vi "Begin Transaction.vi"(8 "error in (no error)":errorcluster, 11 "Sqlite Database Manager in":refnum<class "Sqlite Database Manager.lvclass">) -> (0 "error out":errorcluster, 3 "Sqlite Database Manager out":refnum<class "Sqlite Database Manager.lvclass">)   [LabVIEW 2019, in "HierDAL Library.lvlib" / "Database.lvlib" / "Sqlite Database Manager.lvclass"]
uses:
  Sqlite Database Manager.lvclass
  Sqlite Database Manager.lvclass/Sqlite Database Manager.ctl
  System.Data.SQLite
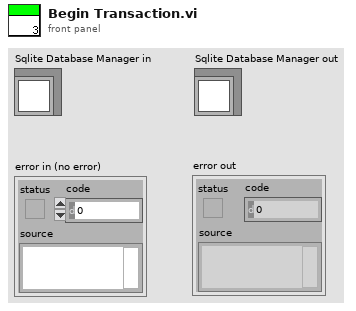
[diagram p1: front panel]
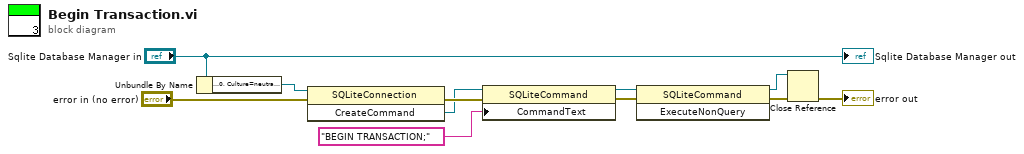
[diagram p0: block diagram]
diagram:
  n1 = Unbundle By Name("Sqlite Database Manager in") -> ("Connection"=w9:refnum<k24>)
  n2 = invoke class="SQLiteConnection" method="CreateCommand"(reference=w9, error in="error in (no error)") -> (error out=w8:errorcluster, "CreateCommand"=w7:refnum<k24>)  [unwired: 1 in, 1 out]
  n3 = property class="SQLiteCommand"(reference=w7, error in=w8, "CommandText"="BEGIN TRANSACTION;") -> (reference out=w4:refnum<k24>, error out=w5:errorcluster)
  n4 = invoke class="SQLiteCommand" method="ExecuteNonQuery"(reference=w4, error in=w5) -> (reference out=w2:refnum<k24>, error out=w3:errorcluster)  [unwired: 1 in, 1 out]
  n5 = Close Reference(reference=w2, error in (no error)=w3) -> (error out=→"error out":errorcluster)
  "Sqlite Database Manager out" <- "Sqlite Database Manager in"
